vi "TeleopEIO.vi"(8 "AnalogIoObjects":T9, 9 "DigitalIoObjects":T23, 10 "Match Info":T24={"Autonomous Elapsed Seconds"=0.0, "TeleOp Elapsed Seconds"=0.0, "Disabled Elapsed Seconds"=0.0, "Visited Autonomous"=FALSE, "Visited TeleOp"=FALSE, "Visited Disabled"=FALSE, "Autonomous Settings"={"Autonomous Style"=enum."Independent", "VI Refnum"=refnum}}, 11 "Call Context":T25) -> ()   [LabVIEW 2015]
doc: "This VI is called for each TeleOp packet received from the DS where the robot is not disabled. It is often used to read from the joysticks and update I/O or to update setpoints for timed control loops. It should complete and return within 20 milliseconds or it may miss DS packets."
uses:
  <vilib>/Rock Robotics/WPI/DriverStation/WPI_DriverStationDerivedRobotMode.ctl
  <vilib>/Rock Robotics/WPI/DriverStation/WPI_DriverStationMatch Info.ctl
  <vilib>/Rock Robotics/WPI/MotorControl/WPI_MotorControlDeviceRef.ctl
  <vilib>/Rock Robotics/WPI/MotorControl/WPI_MotorControlType.ctl
  <vilib>/Rock Robotics/SystemInterfaces/DIO/FPGA_DIOPWMChannel.ctl
  <vilib>/Rock Robotics/WPI/PWM/WPI_PWMDeadband.ctl
  <vilib>/Rock Robotics/WPI/CAN/Jaguar/SubVIs/WPI_CANJaguar_ControlMode.ctl
  <vilib>/Rock Robotics/WPI/CAN/TalonSRX/WPI_CANTalonSRX_APIControlMode.ctl
  <vilib>/Rock Robotics/WPI/DigitalInput/WPI_DigitalInputDevRef.ctl
  <vilib>/Rock Robotics/SystemInterfaces/DIO/FPGA_DIOChannel.ctl
  <vilib>/Rock Robotics/WPI/DigitalOutput/WPI_DigitalOutputDevRef.ctl
  <vilib>/Rock Robotics/WPI/Encoder/WPI_EncoderDevRef.ctl
  <vilib>/Rock Robotics/SystemInterfaces/Encoder/FPGA_EncoderIdx.ctl
  <vilib>/Rock Robotics/SystemInterfaces/Counter/FPGA_CounterCtrSystemIndex.ctl
  <vilib>/Rock Robotics/WPI/Encoder/WPI_EncoderType.ctl
  <vilib>/Rock Robotics/WPI/AnalogChannel/WPI_AnalogChannelDevRef.ctl
  <vilib>/Rock Robotics/SystemInterfaces/AI/FPGA_AIChannel.ctl
  <vilib>/Rock Robotics/SystemInterfaces/AnalogTrigger/FPGA_AnalogTriggerDevRef.ctl
  <vilib>/Rock Robotics/SystemInterfaces/AnalogTrigger/FPGA_AnalogTriggerIndex.ctl
  <vilib>/Rock Robotics/WPI/Counter/WPI_CounterDevRef.ctl
  <vilib>/Rock Robotics/WPI/AnalogOutput/WPI_AOChannelDevRef.ctl
  <vilib>/Rock Robotics/WPI/AnalogOutput/WPI_AnalogOutputChannel.ctl
  <vilib>/Rock Robotics/WPI/Utilities/WPI_GetSetVariantRefNum.vi
  <vilib>/Rock Robotics/Network Tables/SD Write Boolean Array.vi
  <vilib>/Rock Robotics/Network Tables/SD Write Numeric Array.vi
  <vilib>/Rock Robotics/Network Tables/SD Write Boolean.vi
  <vilib>/Rock Robotics/Network Tables/SD Write Number.vi
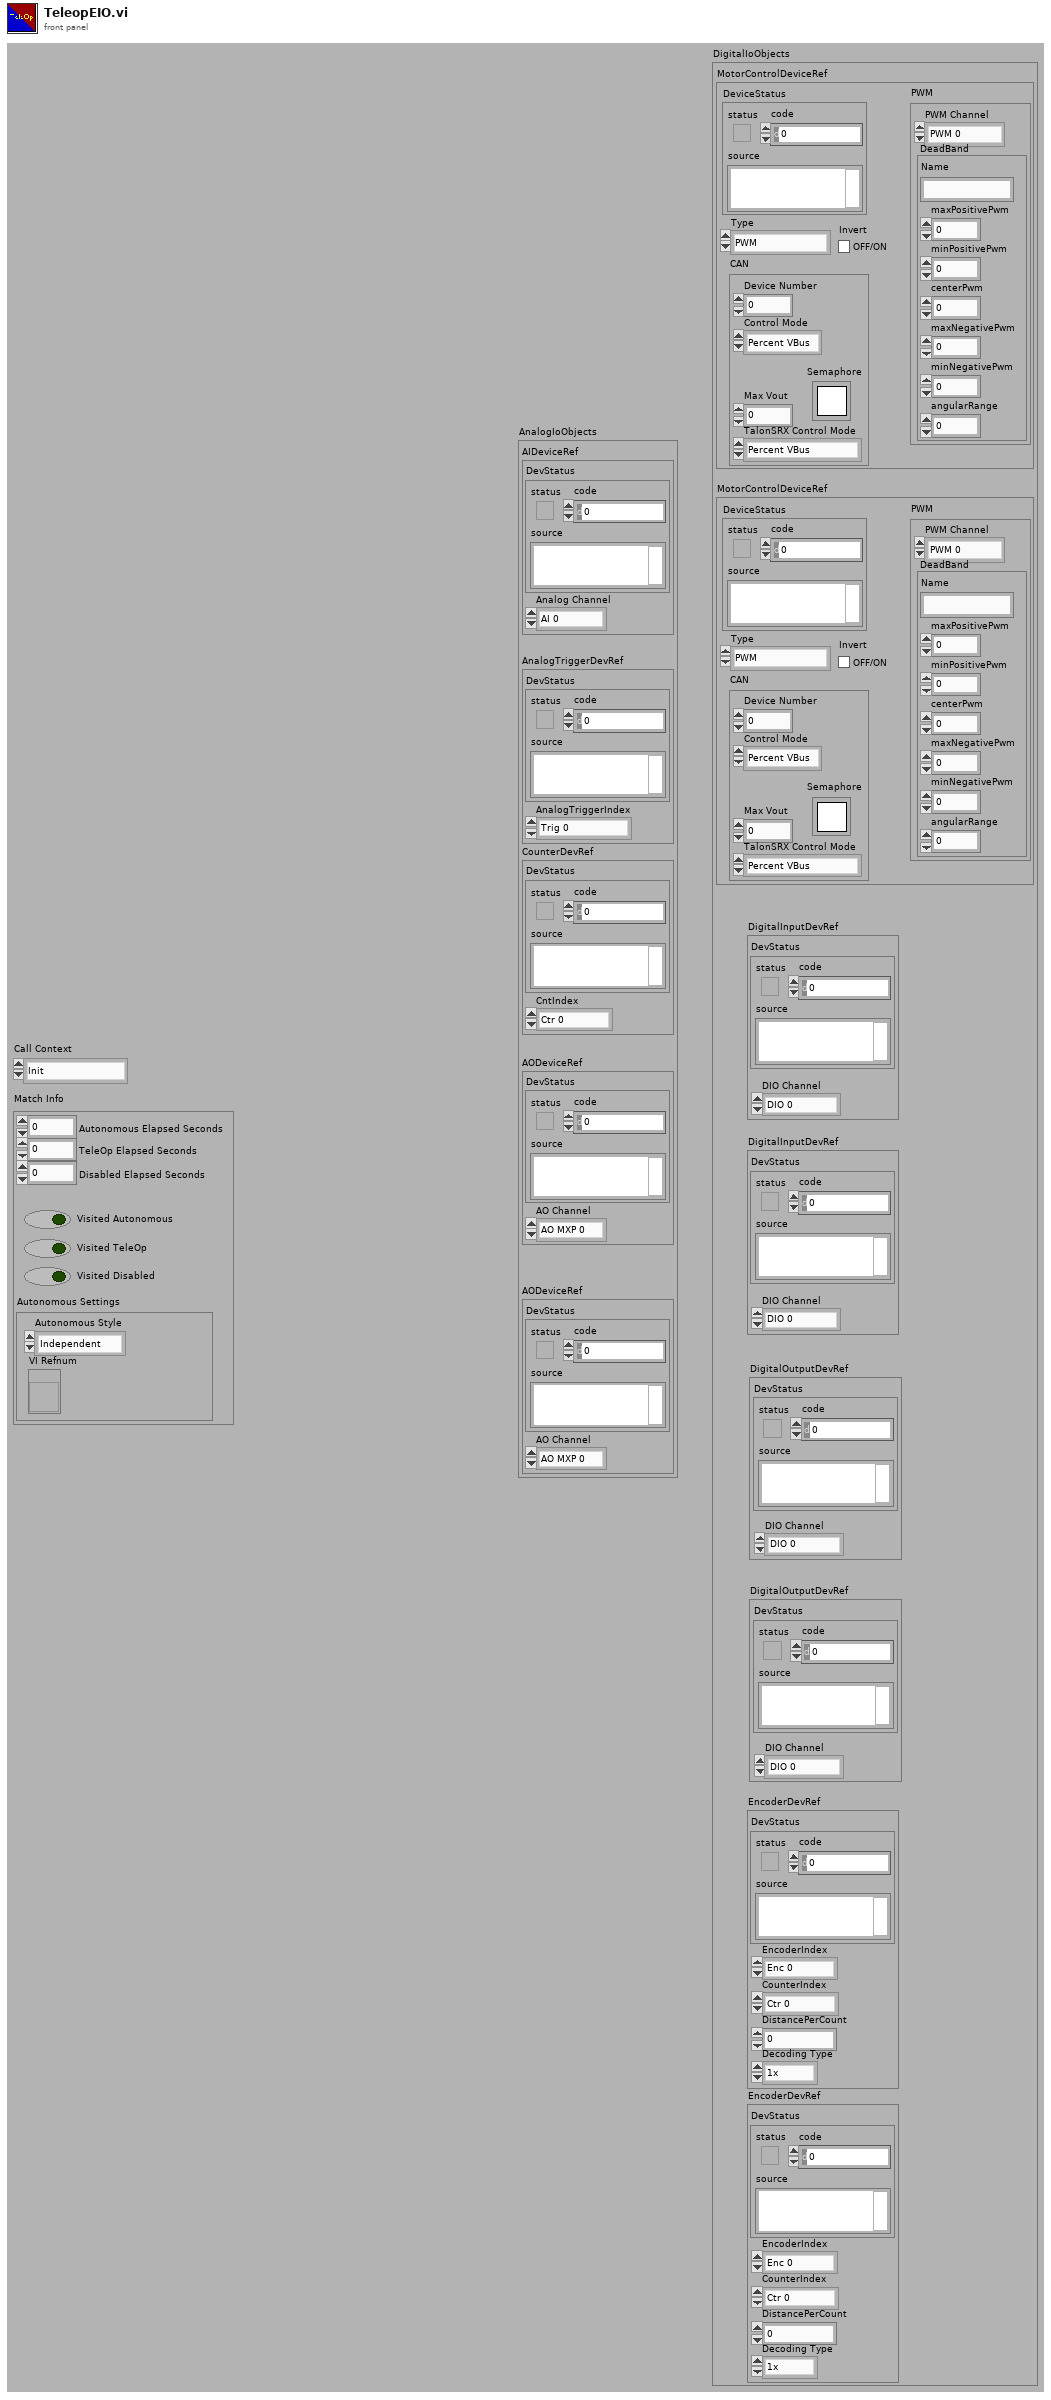
[diagram p1: front panel]
types:
  T1 = typedef "WPI_AnalogChannelDevRef.ctl" = cluster{"DevStatus":errorcluster, "Analog Channel":T2}
  T2 = typedef "FPGA_AIChannel.ctl" = enum8{"AI 0", "AI 1", "AI 2", "AI 3", "AI MXP 0", "AI MXP 1", "AI MXP 2", "AI MXP 3", "Invalid"}
  T3 = typedef "FPGA_AnalogTriggerDevRef.ctl" = cluster{"DevStatus":errorcluster, "AnalogTriggerIndex":T4}
  T4 = typedef "FPGA_AnalogTriggerIndex.ctl" = enum8{"Trig 0", "Trig 1", "Trig 2", "Trig 3", "Trig 4", "Trig 5", "Trig 6", "Trig 7", "Invalid"}
  T5 = typedef "WPI_CounterDevRef.ctl" = cluster{"DevStatus":errorcluster, "CntIndex":T6}
  T6 = typedef "FPGA_CounterCtrSystemIndex.ctl" = enum8{"Ctr 0", "Ctr 1", "Ctr 2", "Ctr 3", "Ctr 4", "Ctr 5", "Ctr 6", "Ctr 7", "Invalid"}
  T7 = typedef "WPI_AOChannelDevRef.ctl" = cluster{"DevStatus":errorcluster, "AO Channel":T8}
  T8 = typedef "WPI_AnalogOutputChannel.ctl" = enum8{"AO MXP 0", "AO MXP 1", "Invalid"}
  T9 = cluster{"AIDeviceRef":T1, "AnalogTriggerDevRef":T3, "CounterDevRef":T5, "AODeviceRef":T7, "AODeviceRef":T7}
  T10 = typedef "WPI_MotorControlDeviceRef.ctl" = cluster{"DeviceStatus":errorcluster, "Type":T11, "PWM":cluster{"PWM Channel":T12, "DeadBand":T13}, "CAN":cluster{"Device Number":u8, "Control Mode":T14, "Semaphore":T15, "Max Vout":dbl, "TalonSRX Control Mode":T16}, "Invert":bool}
  T11 = typedef "WPI_MotorControlType.ctl" = enum16{"PWM", "CAN", "CANTalonSRX"}
  T12 = typedef "FPGA_DIOPWMChannel.ctl" = enum8{"PWM 0", "PWM 1", "PWM 2", "PWM 3", "PWM 4", "PWM 5", "PWM 6", "PWM 7", "PWM 8", "PWM 9", "PWM MXP 0", "PWM MXP 1", "PWM MXP 2", "PWM MXP 3", "PWM MXP 4", "PWM MXP 5", "PWM MXP 6", "PWM MXP 7", "PWM MXP 8", "PWM MXP 9", "Invalid"}
  T13 = typedef "WPI_PWMDeadband.ctl" = cluster{"Name":string, "maxPositivePwm":i32, "minPositivePwm":i32, "centerPwm":i32, "maxNegativePwm":i32, "minNegativePwm":i32, "angularRange":u16}
  T14 = typedef "WPI_CANJaguar_ControlMode.ctl" = enum8{"Percent VBus", "Current", "Speed", "Position", "Voltage"}
  T15 = typedef "Semaphore RefNum" = refnum<k1>
  T16 = typedef "WPI_CANTalonSRX_APIControlMode.ctl" = enum8{"Percent VBus", "Speed", "Position", "Slave", "Unchanged / Invalid", "Voltage Compensation", "Current", "Motion Profile"}
  T17 = typedef "WPI_DigitalInputDevRef.ctl" = cluster{"DevStatus":errorcluster, "DIO Channel":T18}
  T18 = typedef "FPGA_DIOChannel.ctl" = enum8{"DIO 0", "DIO 1", "DIO 2", "DIO 3", "DIO 4", "DIO 5", "DIO 6", "DIO 7", "DIO 8", "DIO 9", "DIO MXP 0", "DIO MXP 1", "DIO MXP 2", "DIO MXP 3", "DIO MXP 4", "DIO MXP 5", "DIO MXP 6", "DIO MXP 7", "DIO MXP 8", "DIO MXP 9", "DIO MXP 10", "DIO MXP 11", "DIO MXP 12", "DIO MXP 13", "DIO MXP 14", "DIO MXP 15", "Invalid"}
  T19 = typedef "WPI_DigitalOutputDevRef.ctl" = cluster{"DIO Channel":T18, "DevStatus":errorcluster}
  T20 = typedef "WPI_EncoderDevRef.ctl" = cluster{"DevStatus":errorcluster, "EncoderIndex":T21, "CounterIndex":T6, "DistancePerCount":dbl, "Decoding Type":T22}
  T21 = typedef "FPGA_EncoderIdx.ctl" = enum8{"Enc 0", "Enc 1", "Enc 2", "Enc 3", "Enc 4", "Enc 5", "Enc 6", "Enc 7", "Invalid"}
  T22 = typedef "WPI_EncoderType.ctl" = enum16{"1x", "2x", "4x"}
  T23 = cluster{"MotorControlDeviceRef":T10, "MotorControlDeviceRef":T10, "DigitalInputDevRef":T17, "DigitalInputDevRef":T17, "DigitalOutputDevRef":T19, "DigitalOutputDevRef":T19, "EncoderDevRef":T20, "EncoderDevRef":T20}
  T24 = typedef "WPI_DriverStationMatch Info.ctl" = cluster{"Autonomous Elapsed Seconds":dbl, "TeleOp Elapsed Seconds":dbl, "Disabled Elapsed Seconds":dbl, "Visited Autonomous":bool, "Visited TeleOp":bool, "Visited Disabled":bool, "Autonomous Settings":cluster{"Autonomous Style":enum16{"Iterative", "Independent"}, "VI Refnum":refnum<vi>}}
  T25 = typedef "WPI_DriverStationDerivedRobotMode.ctl" = enum16{"Init", "Execute", "Stop"}
  T26 = typedef "WPI_JoystickDevRef.ctl" = cluster{"Device":T27}
  T27 = typedef "WPI_JoystickDeviceEnum.ctl" = enum16{"USB 0", "USB 1", "USB 2", "USB 3", "USB 4", "USB 5"}
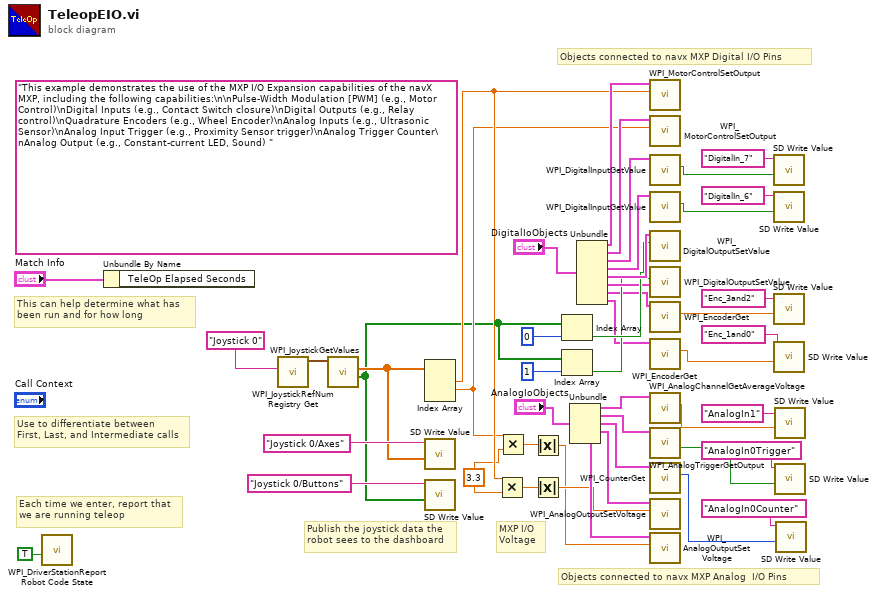
[diagram p0: block diagram]
diagram:
  w5 = 3.3
  (unwired) "This example demonstrates the use of the MXP I/O Expansion capabilities of the navX MXP, including the following capabilities:\n\nPulse-Width Modulation [PWM] (e.g., Motor Control)\nDigital Inputs (e.g., Contact Switch closure)\nDigital Outputs (e.g., Relay control)\nQuadrature Encoders (e.g., Wheel Encoder)\nAnalog Inputs (e.g., Ultrasonic Sensor)\nAnalog Input Trigger (e.g., Proximity Sensor trigger)\nAnalog Trigger Counter\nAnalog Output (e.g., Constant-current LED, Sound) "
  # "Objects connected to navx MXP Analog  I/O Pins"
  # "Objects connected to navx MXP Digital I/O Pins"
  # "MXP I/O\nVoltage"
  # "Publish the joystick data the\nrobot sees to the dashboard"
  # "Each time we enter, report that\nwe are running teleop"
  # "Use to differentiate between\nFirst, Last, and Intermediate calls"
  # "This can help determine what has\nbeen run and for how long"
  n1 = call <vilib>:"WPI_DriverStationReport Robot Code State.vi"("TeleOp"=TRUE ("Autonomous")) -> ()  [unwired: 10 in, 1 out]
  n2 = Unbundle By Name("Match Info") -> ()  [unwired: 1 out]
  n3 = call <vilib>:"WPI_JoystickRefNum Registry Get.vi"("refnum name"="Joystick 0") -> ("JoystickDevRef"=w45:T26)  [unwired: 1 in, 9 out]
  n4 = call <vilib>:"WPI_JoystickGetValues.vi"("JoystickDevRef"=w45) -> ("Buttons"=w29:bool[], "Axes"=w41:dbl[])  [unwired: 6 in, 3 out]
  n5 = Index Array(array=w41) -> (element #1=w31:dbl, element #2=w30:dbl)  [unwired: 3 in, 1 out]
  n6 = call-poly <vilib>:"SD Write Value.vi"("Numeric Array"=w41, "Name"="Joystick 0/Axes") -> ()  [unwired: 8 in, 2 out]
  n7 = call-poly <vilib>:"SD Write Value.vi"("Boolean Array"=w29, "Name"="Joystick 0/Buttons") -> ()  [unwired: 8 in, 2 out]
  n8 = Multiply(x=w31, y=w5) -> (x*y=w4:dbl)
  n9 = Multiply(x=w30, y=w5) -> (x*y=w3:dbl)
  n10 = Absolute Value(x=w3) -> (abs(x)=w1:dbl)
  n11 = Absolute Value(x=w4) -> (abs(x)=w2:dbl)
  n12 = Index Array(array=w29, index=0) -> (element=w34:bool)
  n13 = Index Array(array=w29, index=1) -> (element=w32:bool)
  n14 = Unbundle("AnalogIoObjects") -> ("AIDeviceRef"=w17:T1, "AnalogTriggerDevRef"=w12:T3, "CounterDevRef"=w11:T5, "AODeviceRef"=w13:T7)  [unwired: 1 out]
  n15 = Unbundle("DigitalIoObjects") -> ("MotorControlDeviceRef"=w38:T10, "MotorControlDeviceRef"=w37:T10, "DigitalInputDevRef"=w28:T17, "DigitalInputDevRef"=w23:T17, "DigitalOutputDevRef"=w36:T19, "DigitalOutputDevRef"=w33:T19, "EncoderDevRef"=w22:T20, "EncoderDevRef"=w21:T20)
  n16 = call <vilib>:"WPI_MotorControlSetOutput.vi"("Output"=w31, "MotorControlDevRef"=w38) -> ()  [unwired: 7 in, 3 out]
  n17 = call <vilib>:"WPI_MotorControlSetOutput.vi"("Output"=w30, "MotorControlDevRef"=w37) -> ()  [unwired: 7 in, 3 out]
  n18 = call <vilib>:"WPI_DigitalInputGetValue.vi"("DigitalInputDevRef"=w28) -> ("Value"=w27:bool)  [unwired: 8 in, 2 out]
  n19 = call <vilib>:"WPI_DigitalInputGetValue.vi"("DigitalInputDevRef"=w23) -> ("Value"=w25:bool)  [unwired: 8 in, 2 out]
  n20 = call <vilib>:"WPI_DigitalOutputSetValue.vi"("Value"=w34, "DigitalOutputDevRef"=w36) -> ()  [unwired: 8 in, 2 out]
  n21 = call <vilib>:"WPI_DigitalOutputSetValue.vi"("Value"=w32, "DigitalOutputDevRef"=w33) -> ()  [unwired: 8 in, 2 out]
  n22 = call <vilib>:"WPI_EncoderGet.vi"("EncoderDevRef"=w22) -> ("Distance"=w20:dbl)  [unwired: 5 in, 5 out]
  n23 = call <vilib>:"WPI_EncoderGet.vi"("EncoderDevRef"=w21) -> ("Distance"=w6:dbl)  [unwired: 5 in, 5 out]
  n24 = call <vilib>:"WPI_AnalogChannelGetAverageVoltage.vi"("AIDeviceRef"=w17) -> ("Voltage"=w15:dbl)  [unwired: 8 in, 2 out]
  n25 = call <vilib>:"WPI_AnalogTriggerGetOutput.vi"("AnalogTriggerDevRef"=w12) -> ("Trigger State"=w9:bool)  [unwired: 7 in, 3 out]
  n26 = call <vilib>:"WPI_CounterGet.vi"("CounterDevRef in"=w11) -> ("Value"=w7:i32)  [unwired: 5 in, 5 out]
  n27 = call <vilib>:"WPI_AnalogOutputSetVoltage.vi"("Voltage"=w2, "AODeviceRef"=w13) -> ()  [unwired: 8 in, 2 out]
  n28 = call <vilib>:"WPI_AnalogOutputSetVoltage.vi"("Voltage"=w1, "AODeviceRef"=w13) -> ()  [unwired: 8 in, 2 out]
  n29 = call-poly <vilib>:"SD Write Value.vi"("Boolean"=w27, "Name"="DigitalIn_7") -> ()  [unwired: 8 in, 2 out]
  n30 = call-poly <vilib>:"SD Write Value.vi"("Boolean"=w25, "Name"="DigitalIn_6") -> ()  [unwired: 8 in, 2 out]
  n31 = call-poly <vilib>:"SD Write Value.vi"("Numeric"=w20, "Name"="Enc_3and2") -> ()  [unwired: 8 in, 2 out]
  n32 = call-poly <vilib>:"SD Write Value.vi"("Numeric"=w6, "Name"="Enc_1and0") -> ()  [unwired: 8 in, 2 out]
  n33 = call-poly <vilib>:"SD Write Value.vi"("Numeric"=w15, "Name"="AnalogIn1") -> ()  [unwired: 8 in, 2 out]
  n34 = call-poly <vilib>:"SD Write Value.vi"("Boolean"=w9, "Name"="AnalogIn0Trigger") -> ()  [unwired: 8 in, 2 out]
  n35 = call-poly <vilib>:"SD Write Value.vi"("Numeric"=w7, "Name"="AnalogIn0Counter") -> ()  [unwired: 8 in, 2 out]
